vi "Fetch.vi"(6 "error in (no error)":errorcluster, 9 "VISA resource name":refnum<visa-resource-name>) -> (0 "error out":errorcluster, 2 "Read Buffer":string, 3 "VISA resource name out":refnum<visa-resource-name>)   [LabVIEW 2011, in "Ocean Server OS4000.lvlib"]
doc: "Reads the contents of entire buffer."
uses:
  Ocean Server OS4000.lvlib
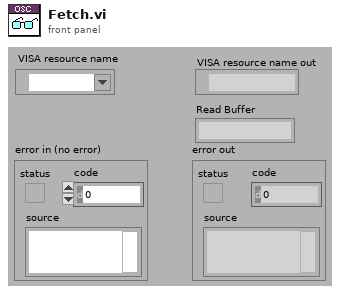
[diagram p1: front panel]
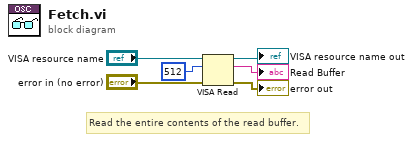
[diagram p0: block diagram]
diagram:
  # "Read the entire contents of the read buffer."
  n1 = VISA Read(VISA resource name="VISA resource name", byte count=u32 512 ("y"), error in (no error)="error in (no error)") -> (VISA resource name out=→"VISA resource name out":refnum<visa-resource-name>, read buffer=→"Read Buffer":string, error out=→"error out":errorcluster)  [unwired: 1 out]
